vi "User-defined Gate function.vi"(8 "Error In":errorcluster, 9 "User-defined Gate":T1, 11 "t":dbl format="%#_4g") -> (0 "Error Out":errorcluster, 3 "User-defined Gate(t)":dbl format="%#_4g")   [LabVIEW 2019]
doc: "Compute the value G(t) where t is the input time point and User-defined Gate is a cluster of two arrays, [t_i], i = 0, ..., n and [G_i}, i = 0,..., n as:\n1) G(t) = 0 if t < t_0 or t > t_n\n2) G(t) is linearly interpolated in between"
uses:
  XY Plot Data.ctl
  <vilib>/Utility/error.llb/Error Cluster From Error Code.vi
  <vilib>/ErrorRing/Error Ring.xnode
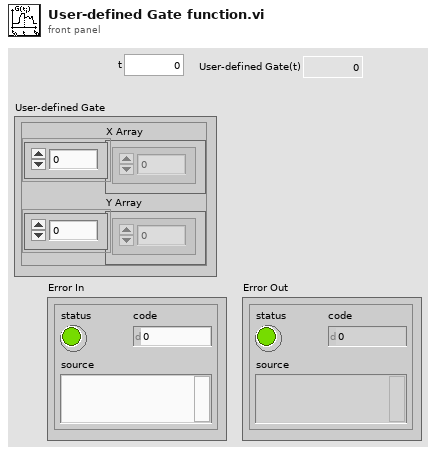
[diagram p1: front panel]
types:
  T1 = typedef "XY Plot Data.ctl" = cluster{"X Array":dbl[], "Y Array":dbl[]}
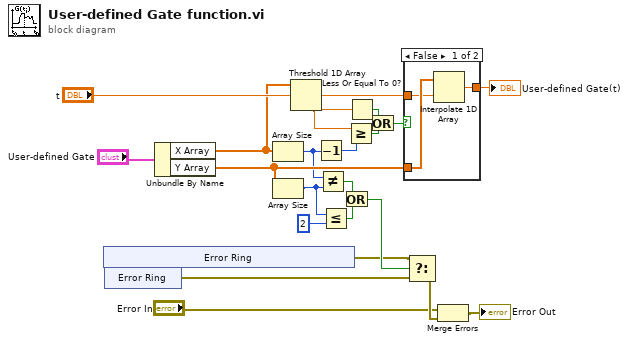
[diagram p0: block diagram]
diagram:
  n1 = xnode "Error Ring"() -> ("error out"=w5:errorcluster)
  n2 = xnode "Error Ring"() -> ("error out"=w4:errorcluster)
  n3 = Unbundle By Name("User-defined Gate") -> ("X Array"=w19:dbl[], "Y Array"=w12:dbl[])
  n4 = Array Size(array=w19) -> (size(s)=w11:i32)
  n5 = Array Size(array=w12) -> (size(s)=w10:i32)
  n6 = Threshold 1D Array(2:"t", 3:w19) -> (0:w18:dbl)  [unwired: 1 in]
  n7 = Decrement(x=w11) -> (x-1=w14:i32)
  n8 = Not Equal?(x=w11, y=w10) -> (x != y?=w8:bool)
  n9 = Less Or Equal?(x=w10, y=2) -> (x <= y?=w7:bool)
  n10 = Or(x=w8, y=w7) -> (x .or. y?=w6:bool)
  n11 = Greater Or Equal?(x=w18, y=w14) -> (x >= y?=w16:bool)
  n12 = Less Or Equal To 0?(x=w18) -> (x <= 0?=w17:bool)
  n13 = Or(x=w17, y=w16) -> (x .or. y?=w15:bool)
  n14 = case shown="False" w15 {
    tunnel: w12 -> [w24 _]
    tunnel: [w23 _] -> w20
    tunnel: w18 -> [w22 _]
    frame False {
      n15 = Interpolate 1D Array(1:w22, 2:w24) -> (0:w23:dbl)
    }
    frame True {
    }
  }
  "User-defined Gate(t)" <- w20
  n16 = Select(t=w5, s=w6, f=w4) -> (s? t:f=w3:errorcluster)
  n17 = Merge Errors("Error In", w3) -> (→"Error Out":errorcluster)
